vi "DontKnow.vi"(8 "error in (no error)":errorcluster, 10 "Array":refnum<class "Configurable Device.lvclass">[](array[class]), 11 "Controller in":refnum<class "Controller.lvclass">) -> (0 "error out":errorcluster, 3 "Controller out":refnum<class "Controller.lvclass">)   [LabVIEW 2014, in "Controller.lvlib" / "Controller.lvclass"]
uses:
  Controller.lvclass
  reusable/DAQ Device/Device/Device.lvclass
  Update Controller Data MSG.lvclass
  Messages/Device Init CVT/Device Init CVT MSG.lvclass
  reusable/Session APIs/File Access/Config Data/Config Data.lvclass
  Messages/Update Device Configuration MSG/Update Device Configuration MSG.lvclass
  Devices/Configurable Device/Configurable Device.lvclass
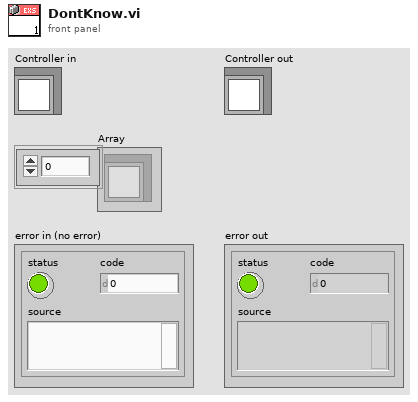
[diagram p1: front panel]
types:
  T1 = typedef "Session - Root.lvclass/Session Handle.ctl" = refnum<data-value>
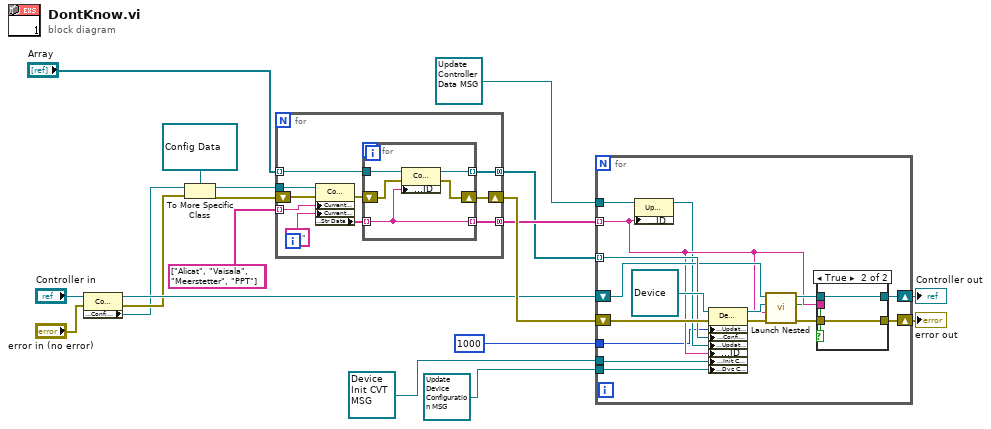
[diagram p0: block diagram]
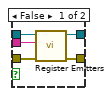
[diagram p2: hidden frame]
diagram:
  (unwired) string[] ["Alicat", "Vaisala", "Meerstetter", "PPT"]
  n1 = property class="Controller"(reference="Controller in", error in="error in (no error)") -> (reference out=w10:refnum<class "Controller.lvclass">, error out=w8:errorcluster, "Accessors:Config Session"=w5:T1)
  n2 = To More Specific Class(target class=refnum<data-value> refnum, reference=w5, error in=w8) -> (specific class reference=w11:refnum<data-value>, error out=w14:errorcluster)
  n3 = for {
    tunnel: string[] ["Alicat", "Vaisala", "Meerstetter", "PPT", "TEC"] -> [w29] mode=indexing
    tunnel: "Array" -> [w26] mode=indexing
    tunnel: w11 -> [w25]
    tunnel: [w24] -> w12 mode=concatenating
    tunnel: [w23] -> w13 mode=concatenating
    shift-right: [w21] -> w15
    shift-left: w14 -> [w22]
    n4 = property class="Config Data"(reference=w25, error in=w22, "Current Section"=w29, "Current Key"="IDs") -> (error out=w20:errorcluster, "Read Array Data:Str Data"=w27:string[])  [unwired: 1 out]
    n5 = for {
      tunnel: w27 -> [w32] mode=indexing
      tunnel: w26 -> [w34]
      tunnel: [w33] -> w24 mode=indexing
      tunnel: [w32] -> w23 mode=indexing
      shift-right: [w31] -> w21
      shift-left: w20 -> [w30]
      n6 = property class="Configurable Device"(reference=w34, error in=w30, "Accessors:ID"=w32) -> (reference out=w33:refnum<class "Configurable Device.lvclass">, error out=w31:errorcluster)
    }
  }
  n7 = for {
    tunnel: w12 -> [w49] mode=indexing
    shift-right: [w42] -> w1
    shift-left: w10 -> [w47]
    tunnel: refnum<class "Update Controller Data MSG.lvclass"> refnum ("Controller.lvlib:Update Data MSG") -> [w48]
    tunnel: w13 -> [w40] mode=indexing
    shift-right: [w41] -> w2
    shift-left: w15 -> [w50]
    tunnel: refnum<class "Device Init CVT MSG.lvclass"> refnum ("Controller.lvlib:Device Init CVT MSG") -> [w38]
    tunnel: refnum<class "Update Device Configuration MSG.lvclass"> refnum ("Controller:Update Device Configuration") -> [w37]
    tunnel: 1000 ("Update Period") -> [w36]
    n8 = property class="Update Data MSG"(reference=w48, "Accessors:ID"=w40) -> (reference out=w39:refnum<class "Update Controller Data MSG.lvclass">)  [unwired: 1 in, 1 out]
    n9 = property class="Device"(reference=refnum<class "Device.lvclass"> refnum ("DAQ Device.lvlib:Device"), error in=w50, "Accessors:Update Period"=w36, "Accessors:Configurable Device"=w49, "Accessors:Update MSG"=w39, "Accessors:ID"=w40, "Accessors:Init CVT MSG"=w38, "Accessors:Dvc Cfg MSG"=w37) -> (reference out=w45:refnum<class "Device.lvclass">, error out=w46:errorcluster)
    n10 = call "Launch Nested.vi"("Error In"=w46, "ID"=w40, "Nested Actor"=w45, "Controller in"=w47) -> ("Error Out"=w43:errorcluster, "Launch Failure?"=w35:bool, "Controller out"=w44:refnum<class "Controller.lvclass">)  [unwired: 5 in]
    n11 = case shown="True" w35 {
      tunnel: w44 -> [w56 w58]
      tunnel: w43 -> [w55 w57]
      tunnel: [w54 w58] -> w42
      tunnel: [w53 w57] -> w41
      tunnel: w40 -> [w52 _]
      frame False {
        n12 = call "Register Emitters.vi"("error in"=w55, "Emitter"=w52, "Controller in"=w56) -> ("error out"=w53:errorcluster, "Controller out"=w54:refnum<class "Controller.lvclass">)  [unwired: 7 in]
      }
      frame True {
      }
    }
  }
  "error out" <- w2
  "Controller out" <- w1
